vi "CVT to JSON.vi"(7 "Select":enum16{"Init", "Get", "Destroy"}(ring), 8 "error in":errorcluster, 11 "cvt in":refnum<data-value>) -> (0 "error out":errorcluster, 2 "json cvt":string, 3 "cvt out":refnum<data-value>)   [LabVIEW 2014, in "CVT.lvclass"]
uses:
  CVT.lvclass
  Controller/Controller.lvclass
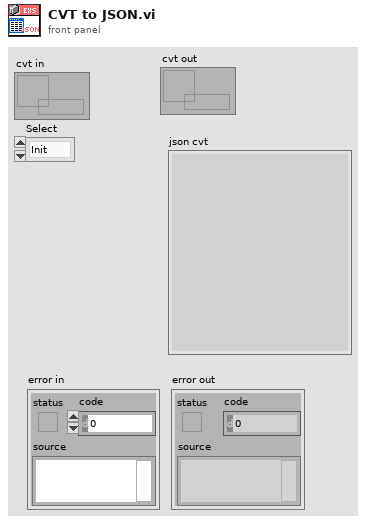
[diagram p1: front panel]
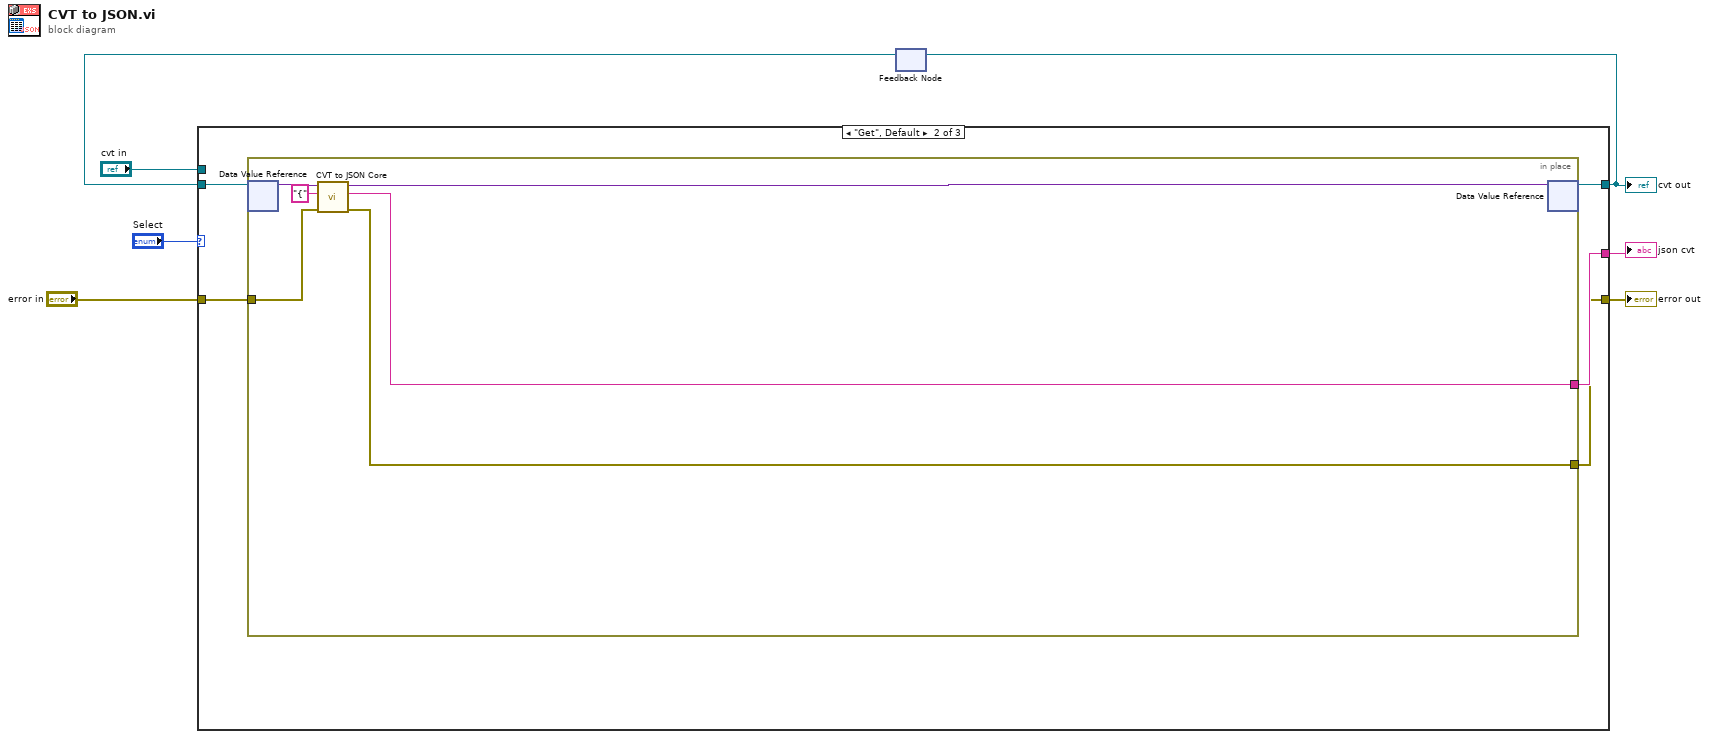
[diagram p0: block diagram]
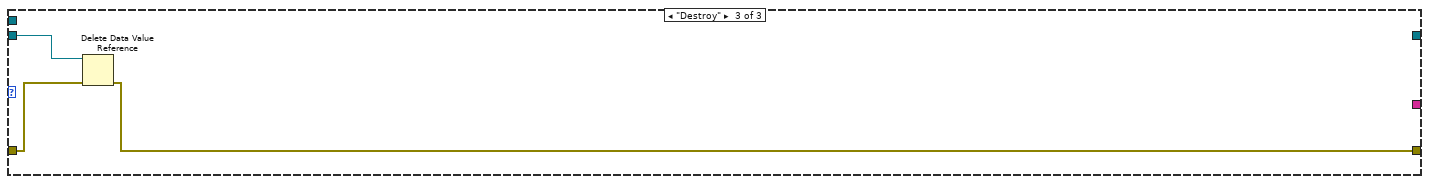
[diagram p3: hidden frame]
diagram:
  n1 = feedback #1() -> (w2:refnum<data-value>)  [unwired: 1 in]
  n2 = case shown="\"Get\", Default" "Select" {
    tunnel: "error in" -> [w9 w14 w22]
    tunnel: [_ w13 _] -> w6
    tunnel: [w9 w12 w21] -> w5
    tunnel: "cvt in" -> [w8 _ _]
    tunnel: [w8 w10 _] -> w1
    tunnel: w2 -> [_ w11 w23]
    frame "Init" {
    }
    frame "Get", Default {
      n3 = in-place {
        in-place-border: [w18] -> w13
        in-place-border: w14 -> [w17]
        in-place-border: [w16] -> w12
        n4 = in-place-dvr #2(w11) -> (w20:variant)  [unwired: 1 out]
        n5 = call "CVT to JSON Core.vi"("error in (no error)"=w17, "StrIn"="{", "variant"=w20) -> ("error out"=w16:errorcluster, "StrOut"=w18:string, "Variant"=w19:variant)  [unwired: 6 in]
        n6 = in-place-dvr #2(w19) -> (w10:refnum<data-value>)  [unwired: 1 out]
      }
    }
    frame "Destroy" {
      n7 = Delete Data Value Reference(data value reference=w23, error in=w22) -> (error out=w21:errorcluster)  [unwired: 1 out]
    }
  }
  "error out" <- w5
  "json cvt" <- w6
  "cvt out" <- w1
  n8 = feedback-in #1(w1) -> ()
